vi "Init.vi"(8 "error in":errorcluster, 11 "PDO Mapping Column Header in":refnum<class "PDO Mapping Column Header.lvclass">) -> (0 "error out":errorcluster, 3 "PDO Mapping Column Header out":refnum<class "PDO Mapping Column Header.lvclass">)   [LabVIEW 2019, in "PDO Grid.lvlib" / "PDO Mapping Column Header.lvclass"]
uses:
  PDO Mapping Column Header.lvclass
  D:/git/Sourcegrid-LabVIEW/source/Cells/ColumnHeader/Column Header.lvclass
  Sourcegrid-LabVIEW/source/Views/ColumnHeader View/ColumnHeader View.lvclass
  D:/git/Sourcegrid-LabVIEW/source/Views/Cell View/Cell View.lvclass
  Sourcegrid-LabVIEW/source/Cells/ColumnHeader/Column Header.lvclass
  Sourcegrid-LabVIEW/source/Font/Font.lvclass
  Sourcegrid-LabVIEW/source/System.Drawing.Color.ctl
  Sourcegrid-LabVIEW/source/SourceGrid.lvlib
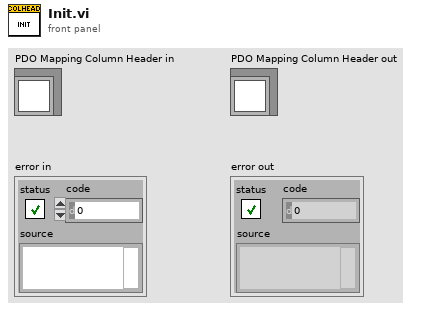
[diagram p1: front panel]
types:
  T1 = typedef "SourceGrid.lvlib/System.Drawing.Color.ctl" = enum16{"AliceBlue", "AntiqueWhite", "Aqua", "Aquamarine", "Azure", "Beige", "Bisque", "Black", "BlanchedAlmond", "Blue", "BlueViolet", "Brown", "BurlyWood", "CadetBlue", "Chartreuse", "Chocolate", "Coral", "CornflowerBlue", "Cornsilk", "Crimson", "Cyan", "DarkBlue", "DarkCyan", "DarkGoldenrod", "DarkGray", "DarkGreen", "DarkKhaki", "DarkMagenta", "DarkOliveGreen", "DarkOrange", "DarkOrchid", "DarkRed", "DarkSalmon", "DarkSeaGreen", "DarkSlateBlue", "DarkSlateGray", "DarkTurquoise", "DarkViolet", "DeepPink", "DeepSkyBlue", "DimGray", "DodgerBlue", "Firebrick", "FloralWhite", "ForestGreen", "Fuchsia", "Gainsboro", "GhostWhite", "Gold", "Goldenrod", "Gray", "Green", "GreenYellow", "Honeydew", "HotPink", "IndianRed", "Indigo", "Ivory", "Khaki", "Lavender", "LavenderBlush", "LawnGreen", "LemonChiffon", "LightBlue", "LightCoral", "LightCyan", "LightGoldenrodYellow", "LightGray", "LightGreen", "LightPink", "LightSalmon", "LightSeaGreen", "LightSkyBlue", "LightSlateGray", "LightSteelBlue", "LightYellow", "Lime", "LimeGreen", "Linen", "Magenta", "Maroon", "MediumAquamarine", "MediumBlue", "MediumOrchid", "MediumPurple", "MediumSeaGreen", "MediumSlateBlue", "MediumSpringGreen", "MediumTurquoise", "MediumVioletRed", "MidnightBlue", "MintCream", "MistyRose", "Moccasin", "NavajoWhite", "Navy", "OldLace", "Olive", "OliveDrab", "Orange", "OrangeRed", "Orchid", "PaleGoldenrod", "PaleGreen", "PaleTurquoise", "PaleVioletRed", "PapayaWhip", "PeachPuff", "Peru", "Pink", "Plum", "PowderBlue", "Purple", "Red", "RosyBrown", "RoyalBlue", "SaddleBrown", "Salmon", "SandyBrown", "SeaGreen", "SeaShell", "Sienna", "Silver", "SkyBlue", "SlateBlue", "SlateGray", "Snow", "SpringGreen", "SteelBlue", "Tan", "Teal", "Thistle", "Tomato", "Transparent", "Turquoise", "Violet", "Wheat", "White", "WhiteSmoke", "Yellow"}
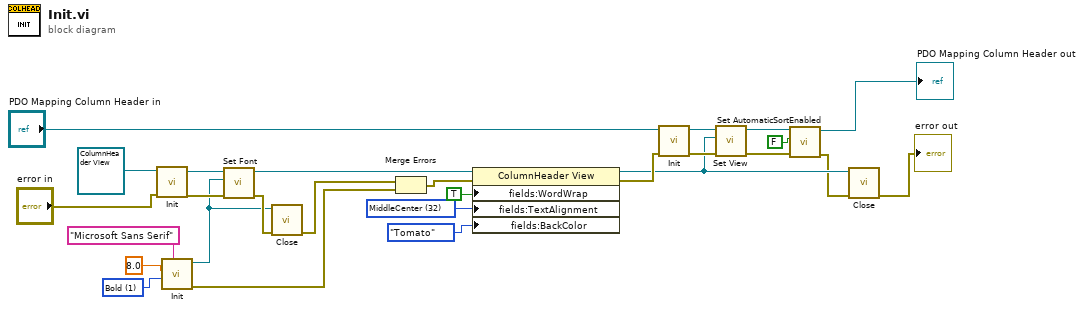
[diagram p0: block diagram]
diagram:
  w17 = 32 items=["TopLeft"=1, "TopCenter"=2, "TopRight"=4, "MiddleLeft"=16, "MiddleCenter"=32, "MiddleRight"=64, "BottomLeft"=256, "BottomCenter"=512, "BottomRight"=1024] ("TextAlignment")
  w22 = 1 items=["Regular"=0, "Bold"=1, "Italic"=2, "Underline"=4, "Strikeout"=8] ("style")
  n1 = call-dynamic "Init.vi"("error in"="error in", "ColumnHeader View in"=refnum<class "ColumnHeader View.lvclass"> refnum ("ColumnHeader View")) -> ("error out"=w19:errorcluster, "ColumnHeader View out"=w25:refnum<class "ColumnHeader View.lvclass">)  [unwired: 8 in]
  n2 = call "Init.vi"("family"="Microsoft Sans Serif", "style"=w22, "emSize"=sgl 8.0) -> ("error out"=w9:errorcluster, "Font out"=w4:refnum<class "Font.lvclass">)  [unwired: 7 in]
  n3 = call-dynamic "Set Font.vi"("error in"=w19, "Font.lvclass"=w4, "View in"=w25) -> ("error out"=w20:errorcluster, "View out"=w21:refnum<class "ColumnHeader View.lvclass">)  [unwired: 7 in]
  n4 = call-dynamic "Close.vi"("error in"=w20, "Font in"=w4) -> ("error out"=w5:errorcluster)  [unwired: 8 in, 1 out]
  n5 = Merge Errors(w5, w9) -> (w16:errorcluster)
  n6 = property class="ColumnHeader View"(reference=w21, error in=w16, "fields:WordWrap"=TRUE ("WordWrap"), "fields:TextAlignment"=w17, "fields:BackColor"=System.Drawing.Color."Tomato" ("Color")) -> (reference out=w3:refnum<class "ColumnHeader View.lvclass">, error out=w13:errorcluster)
  n7 = call-parent "Init.vi"("error in"=w13, "Column Header in"="PDO Mapping Column Header in") -> ("error out"=w27:errorcluster, "Column Header out"=w15:refnum<class "PDO Mapping Column Header.lvclass">)  [unwired: 8 in]
  n8 = call-dynamic "Set View.vi"("error in"=w27, "CellView"=w3, "Cell in"=w15) -> ("error out"=w11:errorcluster, "Cell out"=w12:refnum<class "PDO Mapping Column Header.lvclass">)  [unwired: 7 in]
  n9 = call "Set AutomaticSortEnabled.vi"("error in"=w11, "AutomaticSortEnabled"=FALSE, "ColumnHeader in"=w12) -> ("error out"=w2:errorcluster, "ColumnHeader out"=→"PDO Mapping Column Header out":refnum<class "PDO Mapping Column Header.lvclass">)  [unwired: 7 in]
  n10 = call-dynamic "Close.vi"("error in"=w2, "Cell View in"=w3) -> ("error out"=→"error out":errorcluster)  [unwired: 8 in, 1 out]
